vi "Control Path.vi"(11 "GaugeEditorPanel in":refnum<class "GaugeEditorPanel.lvclass">) -> (2 "Control Paths":path[](array[path]))   [LabVIEW 2020, in "VolatusGUIControls.lvlib" / "GaugeEditorPanel.lvclass"]
uses:
  GaugeEditorPanel.lvclass
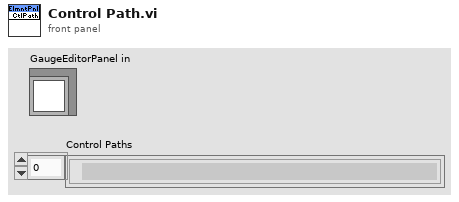
[diagram p1: front panel]
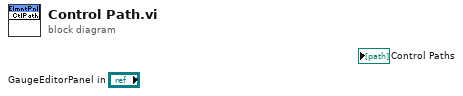
[diagram p0: block diagram]
diagram:
